vi "close_camera.vi"(8 "error in (no error)":errorcluster, 11 ".NET Refnum in":refnum<k24>) -> (0 "error out":errorcluster, 3 ".NET Refnum out":refnum<k24>)   [LabVIEW 2021]
uses:
  C:/Program Files/Thorlabs/Scientific Imaging/ThorCam/uc480DotNet.dll
  Program Files/Thorlabs/Scientific Imaging/ThorCam/uc480DotNet.dll
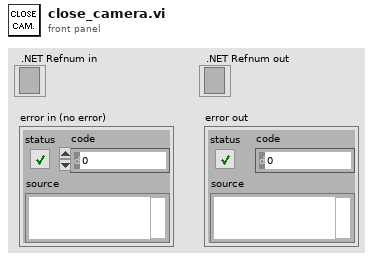
[diagram p1: front panel]
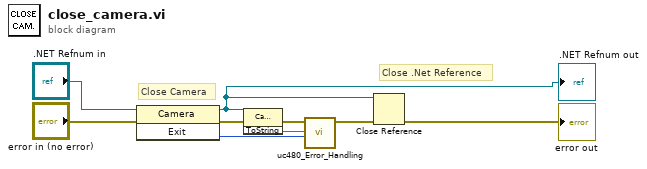
[diagram p0: block diagram]
diagram:
  # "Close .Net Reference"
  # "Close Camera"
  n1 = invoke class="Camera" method="Exit"(reference=".NET Refnum in", error in="error in (no error)") -> (reference out=w7:refnum<k24>, error out=w3:errorcluster, "Exit"=w4:i32)  [unwired: 1 in]
  ".NET Refnum out" <- w7
  n2 = invoke class="Camera" method="ToString"(reference=w7, error in=w3) -> (error out=w2:errorcluster, "ToString"=w1:string)  [unwired: 1 in, 1 out]
  n3 = call "uc480_Error_Handling.vi"("Error Code"=w4, "Error String"=w1, "Error In"=w2) -> ("Error Out"=w5:errorcluster)  [unwired: 8 in]
  n4 = Close Reference ("Close Referenz")(reference=w7, error in (no error)=w5) -> (error out=→"error out":errorcluster)
